vi "Discover Message Type.vi"(9 "Message Enqueuer":refnum<class "Message Enqueuer.lvclass">, 11 "Message in":refnum<class "Message.lvclass">) -> (1 "Message Valid":bool, 3 "Message out":refnum<class "Message.lvclass">)   [LabVIEW 2023, in "Iterator Actor.lvlib" / "Iterator NR Actor.lvclass"]
uses:
  Iterator NR Actor.lvclass
  Iterator NR Actor.lvclass/Iterator NR Actor.ctl
  Iterator NR Actor Messages/Abstract Iteration Msg/Abstract Iteration Msg.lvclass
  <vilib>/ActorFramework/Message/Message.lvclass
  <vilib>/ActorFramework/Message Enqueuer/Message Enqueuer.lvclass
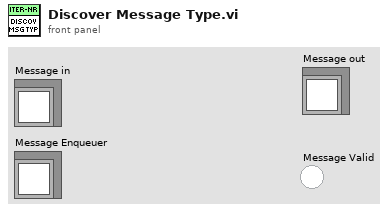
[diagram p1: front panel]
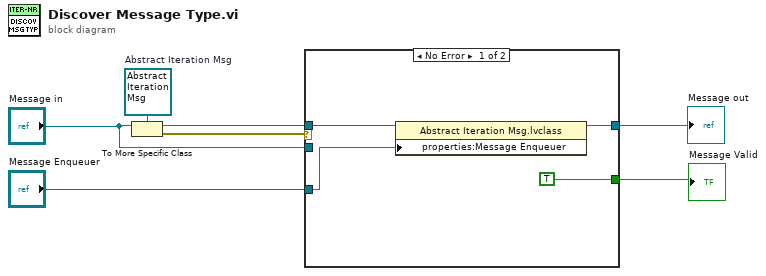
[diagram p0: block diagram]
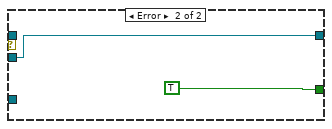
[diagram p2: hidden frame]
diagram:
  w7 = refnum<class "Abstract Iteration Msg.lvclass"> refnum  # Abstract Iteration Msg
  n1 = To More Specific Class(target class=w7, reference="Message in") -> (specific class reference=w4:refnum<class "Abstract Iteration Msg.lvclass">, error out=w6:errorcluster)  [unwired: 1 in]
  n2 = case shown="No Error" w6 {
    tunnel: [TRUE TRUE] -> w5
    tunnel: w4 -> [w10 _]
    tunnel: [w9 w12] -> w2
    tunnel: "Message in" -> [_ w12]
    tunnel: "Message Enqueuer" -> [w8 _]
    frame No Error {
      n3 = property class="Abstract Iteration Msg.lvclass"(reference=w10, "properties:Message Enqueuer"=w8) -> (reference out=w9:refnum<class "Abstract Iteration Msg.lvclass">)  [unwired: 1 in, 1 out]
    }
    frame Error {
    }
  }
  "Message Valid" <- w5
  "Message out" <- w2
